vi "Extract Data Names.vi"(8 "error in (no error)":errorcluster, 11 "Data Cluster":T2) -> (0 "error out":errorcluster, 2 "Task D-O Channels":string[][](array[string]), 3 "output cluster":T2)   [LabVIEW 2018, in "DAQ.lvlib"]
uses:
  DAQ.lvlib
  Acquisition/Task Cluster.ctl
  <resource>/objmgr/daqmx.rc
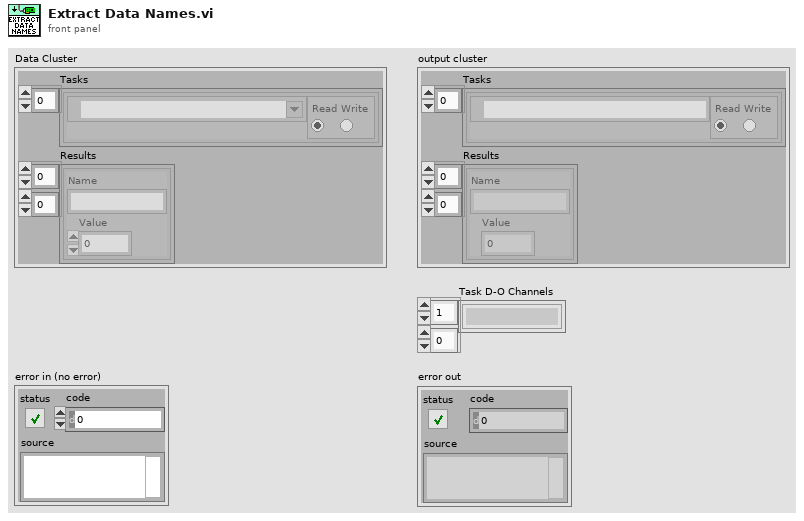
[diagram p1: front panel]
types:
  T1 = typedef "Task Cluster.ctl" = cluster{"DAQmx Task":refnum<k21>, "Read-Write Radio":enum32{"Read", "Write"}}
  T2 = cluster{"Tasks":T1[], "Results":cluster{"Name":string, "Value":dbl}[][]}
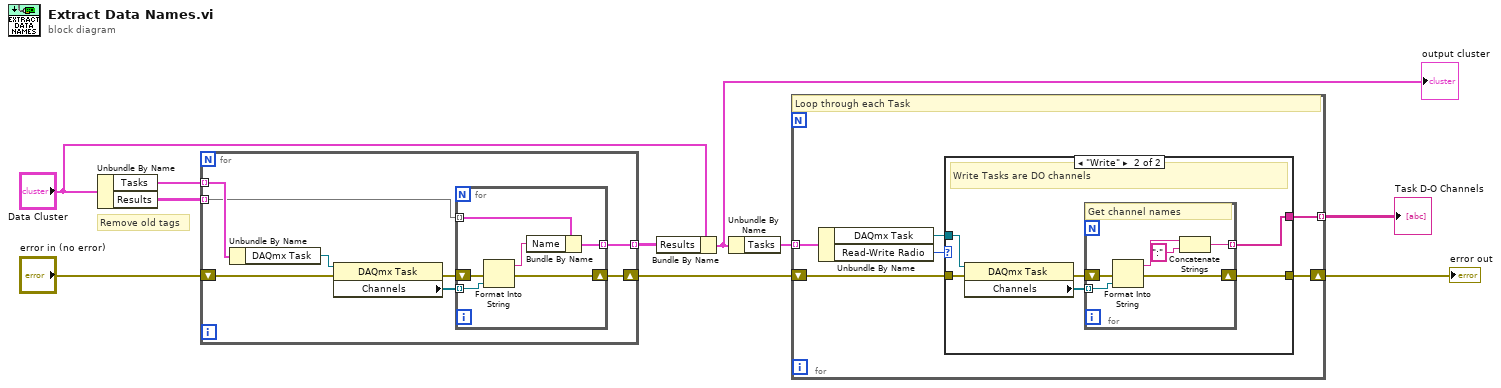
[diagram p0: block diagram]
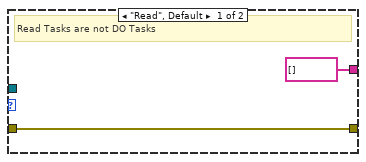
[diagram p2: hidden frame]
diagram:
  # "Remove old tags"
  n1 = Unbundle By Name("Data Cluster") -> ("Tasks"=w6:T1[], "Results"=w7:cluster{"Name":string, "Value":dbl}[][])
  n2 = for {
    tunnel: w6 -> [w18] mode=indexing
    shift-right: [w14] -> w10
    shift-left: "error in (no error)" -> [w17]
    tunnel: w7 -> [w12] mode=indexing
    tunnel: [w11] -> w8 mode=indexing
    n3 = Unbundle By Name(w18) -> ("DAQmx Task"=w16:refnum<k21>)
    n4 = property class="DAQmx Task"(reference=w16, error in=w17) -> (error out=w13:errorcluster, "Channels"=w15:refnum<k21>[])  [unwired: 1 out]
    n5 = for {
      tunnel: w15 -> [w23] mode=indexing
      shift-right: [w24] -> w14
      shift-left: w13 -> [w22]
      tunnel: w12 -> [w21] mode=indexing
      tunnel: [w20] -> w11 mode=indexing
      n6 = Format Into String(error in=w22, w23) -> (resulting string=w19:string, error out=w24:errorcluster)  [unwired: 2 in]
      n7 = Bundle By Name(cluster=w21, "Name"=w19) -> (w20:cluster{"Name":string, "Value":dbl})
    }
  }
  n8 = Bundle By Name(cluster="Data Cluster", "Results"=w8) -> (w5:T2)
  "output cluster" <- w5
  n9 = Unbundle By Name(w5) -> ("Tasks"=w9:T1[])
  n10 = for {
    tunnel: w9 -> [w30] mode=indexing
    shift-right: [w27] -> w2
    shift-left: w10 -> [w25]
    tunnel: [w28] -> w3 mode=indexing
    # "Loop through each Task"
    n11 = Unbundle By Name(w30) -> ("DAQmx Task"=w26:refnum<k21>, "Read-Write Radio"=w29:enum32{"Read", "Write"})
    n12 = case shown="\"Write\"" w29 {
      tunnel: [string[] [] w33] -> w28
      tunnel: [w32 w38] -> w27
      tunnel: w26 -> [_ w37]
      tunnel: w25 -> [w32 w36]
      frame "Read", Default {
        # "Read Tasks are not DO Tasks"
      }
      frame "Write" {
        # "Write Tasks are DO channels"
        n13 = property class="DAQmx Task"(reference=w37, error in=w36) -> (error out=w35:errorcluster, "Channels"=w34:refnum<k21>[])  [unwired: 1 out]
        n14 = for {
          tunnel: w34 -> [w44] mode=indexing
          shift-right: [w42] -> w38
          shift-left: w35 -> [w43]
          tunnel: [w39] -> w33 mode=indexing
          # "Get channel names"
          n15 = Format Into String(error in=w43, w44) -> (resulting string=w41:string, error out=w42:errorcluster)  [unwired: 2 in]
          n16 = Concatenate Strings(w41, ":" ("string")) -> (w39:string)
        }
      }
    }
  }
  "error out" <- w2
  "Task D-O Channels" <- w3
